vi "Find Test Cases.vi"(8 "error in (no error)":errorcluster, 10 "Project or Class Path":path, 11 "Indexing Test Finder In":refnum<class "Indexing Test Finder.lvclass">) -> (0 "error out":errorcluster, 3 "Indexing Test Finder Out":refnum<class "Indexing Test Finder.lvclass">)   [LabVIEW 2020, in "Indexing Test Finder.lvclass"]
uses:
  Indexing Test Finder.lvclass
  Test Finder/Test Finder.lvclass
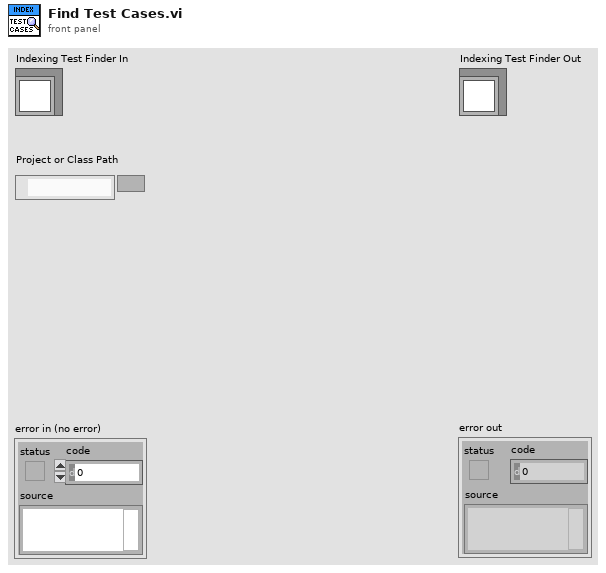
[diagram p1: front panel]
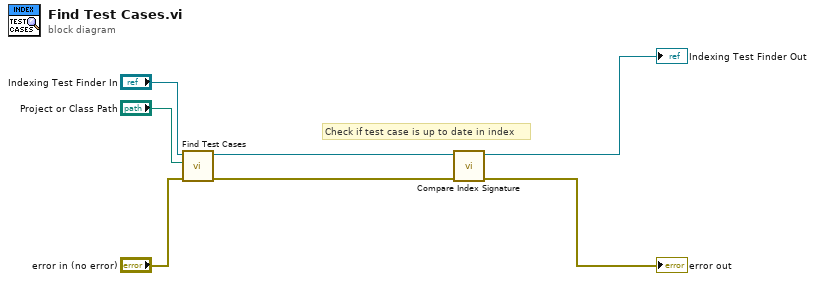
[diagram p0: block diagram]
diagram:
  # "Check if test case is up to date in index"
  n1 = call-parent "Find Test Cases.vi"("error in (no error)"="error in (no error)", "Project or Class Path"="Project or Class Path", "Test Finder In"="Indexing Test Finder In") -> ("error out"=w2:errorcluster, "Test Finder Out"=w4:refnum<class "Indexing Test Finder.lvclass">)  [unwired: 7 in]
  n2 = call "Compare Index Signature.vi"("error in (no error)"=w2, "Indexing Test Finder in"=w4) -> ("error out"=→"error out":errorcluster, "Indexing Test Finder out"=→"Indexing Test Finder Out":refnum<class "Indexing Test Finder.lvclass">)  [unwired: 8 in]
